vi "Get Values.vi"(0 "DVR In":refnum<data-value>, 1 "Subpanel Ref":refnum<vi>, 5 "Status Ref":refnum<vi>, 7 "Config Ref":refnum<vi>, 9 "Mode Ref":refnum<vi>, 11 "Error In":errorcluster) -> (4 "DVR Out":refnum<data-value>, 15 "Error Out":errorcluster)   [LabVIEW 2020, in "Test.lvclass"]
doc: "It will wait for previous called SubVI to get results from it and update it in the DVR"
uses:
  Test.lvclass
  Children/INL DNL Test/INL DNL Test.lvclass
  D:/SDLC/Class/INL DNL Test/Test/Parent/Test.lvclass
  Device/Parent/Device.lvclass
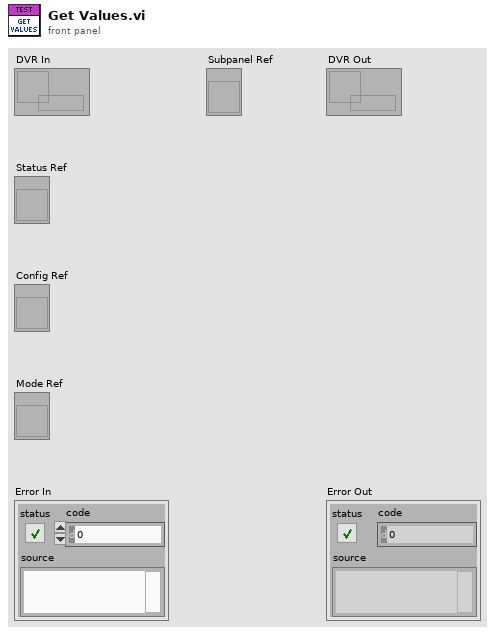
[diagram p1: front panel]
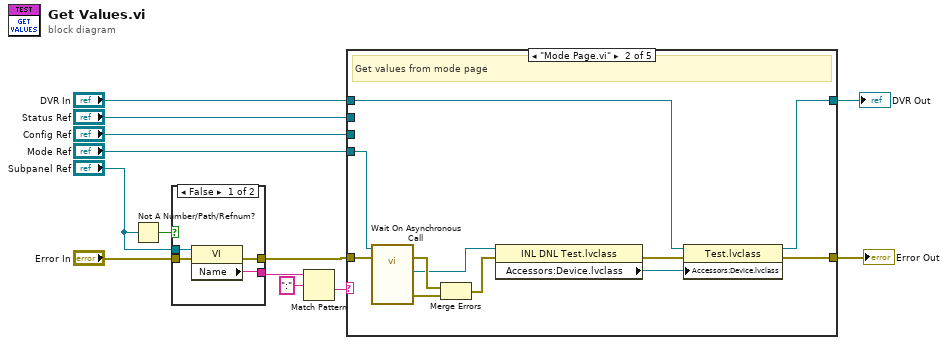
[diagram p0: block diagram]
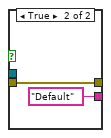
[diagram p2: hidden frame]
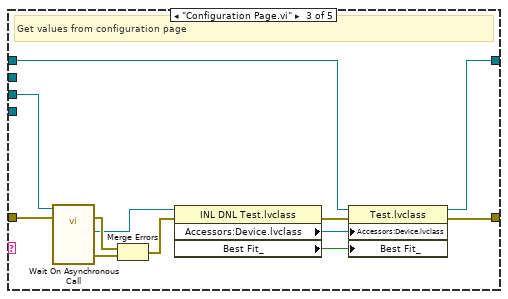
[diagram p4: hidden frame]
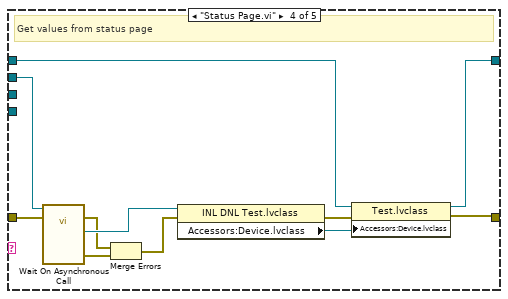
[diagram p5: hidden frame]
diagram:
  n1 = Not A Number/Path/Refnum?(number/path/refnum="Subpanel Ref") -> (NaN/Path/Refnum?=w9:bool)
  n2 = case shown="False" w9 {
    tunnel: "Error In" -> [w17 w19]
    tunnel: [w16 w19] -> w6
    tunnel: [w15 "Default" ("Name")] -> w8
    tunnel: "Subpanel Ref" -> [w14 _]
    frame False {
      n3 = property class="VI"(reference=w14, error in=w17) -> (error out=w16:errorcluster, "Name"=w15:string)  [unwired: 1 out]
    }
    frame True {
    }
  }
  n4 = Match Pattern(string=w8, regular expression=":") -> (after substring=w5:string)  [unwired: 1 in, 3 out]
  n5 = case shown="\"Mode Page.vi\"" w5 {
    tunnel: w6 -> [w21 w32 w41 w55 w57]
    tunnel: [w21 w27 w34 w45 w57] -> w3
    tunnel: "DVR In" -> [w20 w26 w36 w48 w56]
    tunnel: [w20 w23 w35 w46 w56] -> w2
    tunnel: "Mode Ref" -> [_ w31 _ _ _]
    tunnel: "Config Ref" -> [_ _ w40 _ _]
    tunnel: "Status Ref" -> [_ _ _ w54 _]
    frame "Home Page.vi" {
      # "Get values from home page"
    }
    frame "Mode Page.vi" {
      # "Get values from mode page"
      n6 = call-by-ref "Wait On Asynchronous Call"(reference=w31, error in=w32) -> (error out=w30:errorcluster, "Error out"=w29:errorcluster, "INL DNL Test out"=w24:refnum<class "INL DNL Test.lvclass">)  [unwired: 10 in, 1 out]
      n7 = Merge Errors(w30, w29) -> (w28:errorcluster)
      n8 = property class="INL DNL Test.lvclass"(reference=w24, error in=w28) -> (error out=w25:errorcluster, "Accessors:Device.lvclass"=w22:refnum<class "Device.lvclass">)  [unwired: 1 out]
      n9 = property class="Test.lvclass"(reference=w26, error in=w25, "Accessors:Device.lvclass"=w22) -> (reference out=w23:refnum<data-value>, error out=w27:errorcluster)
    }
    frame "Configuration Page.vi" {
      # "Get values from configuration page"
      n10 = call-by-ref "Wait On Asynchronous Call"(reference=w40, error in=w41) -> (error out=w39:errorcluster, "Error out"=w38:errorcluster, "INL DNL Test out"=w37:refnum<class "INL DNL Test.lvclass">)  [unwired: 10 in, 1 out]
      n11 = Merge Errors(w39, w38) -> (w44:errorcluster)
      n12 = property class="INL DNL Test.lvclass"(reference=w37, error in=w44) -> (error out=w43:errorcluster, "Accessors:Device.lvclass"=w42:refnum<class "Device.lvclass">, "Best Fit_"=w33:bool)  [unwired: 1 out]
      n13 = property class="Test.lvclass"(reference=w36, error in=w43, "Accessors:Device.lvclass"=w42, "Best Fit_"=w33) -> (reference out=w35:refnum<data-value>, error out=w34:errorcluster)
    }
    frame "Status Page.vi" {
      # "Get values from status page"
      n14 = call-by-ref "Wait On Asynchronous Call"(reference=w54, error in=w55) -> (error out=w51:errorcluster, "Error out"=w52:errorcluster, "INL DNL Test out"=w53:refnum<class "INL DNL Test.lvclass">)  [unwired: 10 in, 1 out]
      n15 = Merge Errors(w51, w52) -> (w50:errorcluster)
      n16 = property class="INL DNL Test.lvclass"(reference=w53, error in=w50) -> (error out=w49:errorcluster, "Accessors:Device.lvclass"=w47:refnum<class "Device.lvclass">)  [unwired: 1 out]
      n17 = property class="Test.lvclass"(reference=w48, error in=w49, "Accessors:Device.lvclass"=w47) -> (reference out=w46:refnum<data-value>, error out=w45:errorcluster)
    }
    frame Default {
      # "Default state"
    }
  }
  "Error Out" <- w3
  "DVR Out" <- w2
